vi "断电保存全局.vi"() -> ()   [LabVIEW 2016, in "潮位站数据传输.lvlib"]
panel:
  in  "记录报文":bool=TRUE
  in  "数据查表起始时间":T1
  in  "配置信息":T2
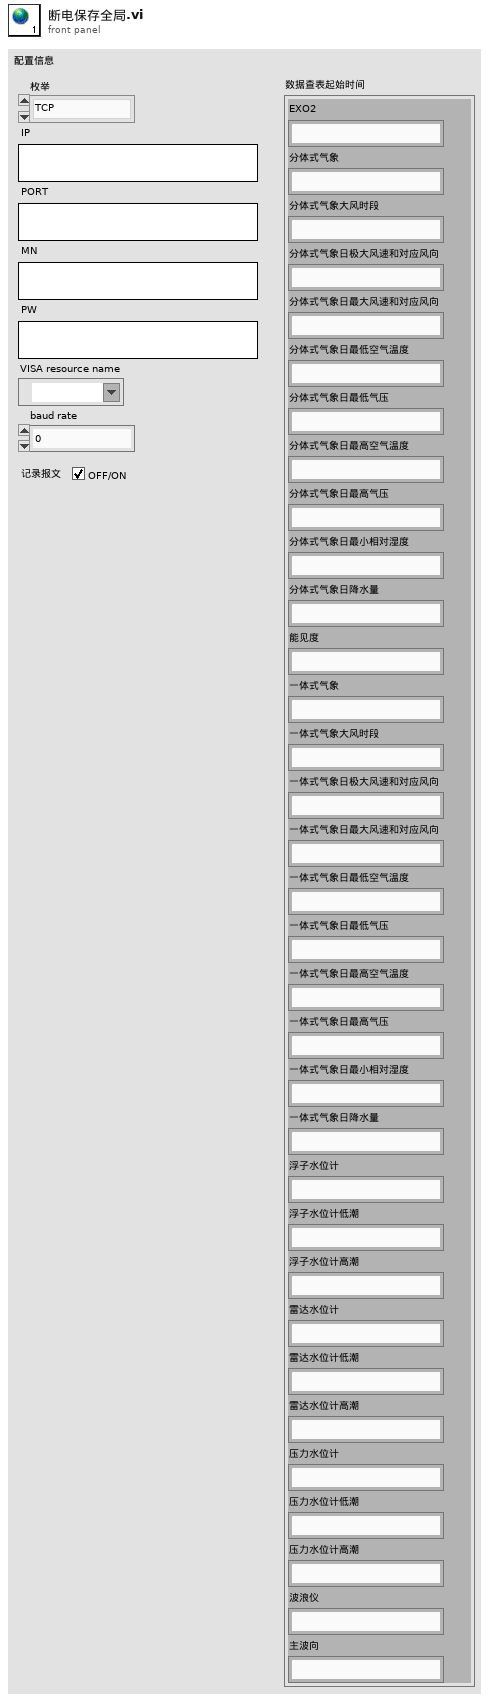
[diagram p1: front panel]
types:
  T1 = cluster{"EXO2":string, "分体式气象":string, "分体式气象大风时段":string, "分体式气象日极大风速和对应风向":string, "分体式气象日最大风速和对应风向":string, "分体式气象日最低空气温度":string, "分体式气象日最低气压":string, "分体式气象日最高空气温度":string, "分体式气象日最高气压":string, "分体式气象日最小相对湿度":string, "分体式气象日降水量":string, "能见度":string, "一体式气象":string, "一体式气象大风时段":string, "一体式气象日极大风速和对应风向":string, "一体式气象日最大风速和对应风向":string, "一体式气象日最低空气温度":string, "一体式气象日最低气压":string, "一体式气象日最高空气温度":string, "一体式气象日最高气压":string, "一体式气象日最小相对湿度":string, "一体式气象日降水量":string, "浮子水位计":string, "浮子水位计低潮":string, "浮子水位计高潮":string, "雷达水位计":string, "雷达水位计低潮":string, "雷达水位计高潮":string, "压力水位计":string, "压力水位计低潮":string, "压力水位计高潮":string, "波浪仪":string, "主波向":string}
  T2 = cluster{"枚举":enum16{"TCP", "serial"}, "IP":string, "PORT":string, "MN":string, "PW":string, "VISA resource name":refnum<visa-resource-name>, "baud rate":u32}
diagram:
